vi "BIN-PAQ-week-GetFolderLocations.vi"(8 "error in (no error)":errorcluster, 9 "Time-End":timestamp, 11 "Time-Start":timestamp) -> (0 "error out":errorcluster, 1 "Overlap?":bool, 3 "Folders":string[](array[string]))   [LabVIEW 2020, in "Sgraph_lib_V1.lvlib" / "DBAL-BIN.lvclass"]
doc: "Find the folders where the historian files are located for the 'per week' pace"
uses:
  DBAL-BIN.lvclass
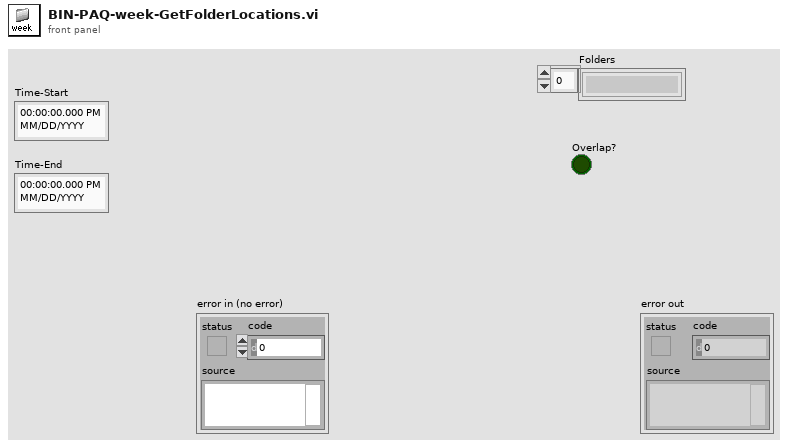
[diagram p1: front panel]
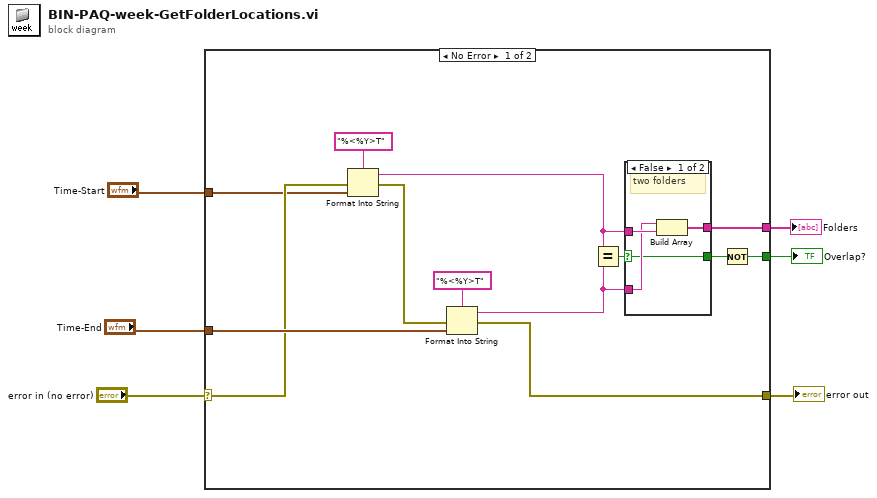
[diagram p0: block diagram]
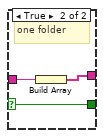
[diagram p2: hidden frame]
diagram:
  n1 = case shown="No Error" "error in (no error)" {
    selector: "error in (no error)" -> [w15 w27]
    tunnel: "Time-Start" -> [w10 _]
    tunnel: "Time-End" -> [w16 _]
    tunnel: [w7 w27] -> w3
    tunnel: [w14 _] -> w2
    tunnel: [w12 _] -> w1
    frame No Error {
      n2 = Format Into String(format string="%<%Y>T", error in=w15, w10) -> (resulting string=w11:string, error out=w8:errorcluster)  [unwired: 1 in]
      n3 = Format Into String(format string="%<%Y>T", error in=w8, w16) -> (resulting string=w9:string, error out=w7:errorcluster)  [unwired: 1 in]
      n4 = Equal?(x=w11, y=w9) -> (x = y?=w17:bool)
      n5 = case shown="False" w17 {
        selector: w17 -> [w20 w24]
        tunnel: w11 -> [w23 w26]
        tunnel: [w21 w25] -> w14
        tunnel: w9 -> [w22 _]
        tunnel: [w20 w24] -> w13
        frame False {
          # "two folders"
          n6 = Build Array(w22, w23) -> (w21:string[])
        }
        frame True {
          # "one folder"
          n7 = Build Array(w26) -> (w25:string[])
        }
      }
      n8 = Not(x=w13) -> (.not. x?=w12:bool)
    }
    frame Error {
    }
  }
  "error out" <- w3
  "Folders" <- w2
  "Overlap?" <- w1
